vi "Instrument.Lockin.AppLauncher.vi"() -> ()   [LabVIEW 2019, in "Instrument.Lockin.lvlib" / "Instrument.Lockin.lvclass"]
uses:
  Instrument.Lockin.lvclass
  Instrument.Lockin.lvclass/Instrument.Lockin.ctl
  Instrument UI.Lockin/Instrument UI.Lockin.lvclass
  <userlib>/_OpenG.lib/appcontrol/appcontrol.llb/openg_application_control.lvlib
  <userlib>/LevyLab/Instrument Framework/Instrument UI/Instrument UI.lvclass
  <userlib>/LevyLab/Instrument Framework/Instrument/Instrument.lvclass
  <vilib>/numeric/Random Number (Range) U64.vi
  <vilib>/JKI/JKI SMO/SMO/Typedefs/SMOState --Enum.ctl
  <vilib>/JKI/JKI SMO/SMO/SMO.lvclass
  <vilib>/JKI/JKI SMO/SMO.UI/SMO.UI.lvclass
  Lockin.Utilities/Lockin.Utilities.lvlib
panel:
  in  "Examine Configuration.ini":bool
  out "error out":errorcluster
  in  "Splash Status":string="Push Start to Start..." caption="String"
  in  "Debug Mode":bool
  in  "Start Application":bool caption="Play"
  in  "Stop Application":bool caption="Stop"
  out "version":string
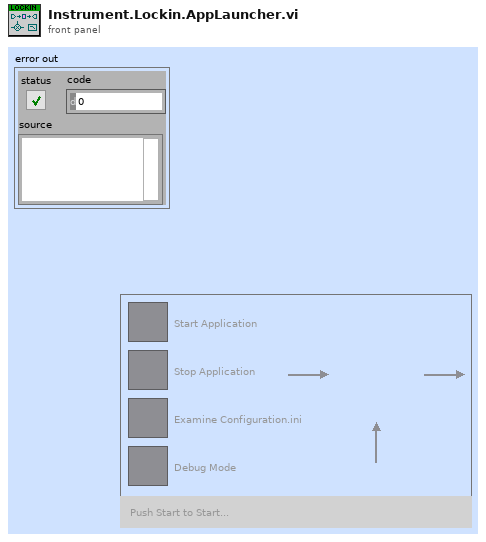
[diagram p1: front panel]
types:
  T1 = typedef "SMO.lvclass/SMOState --Enum.ctl" = enum16{"unknown", "Created", "Started", "Stopped"}
  T2 = enum32{"Invalid", "Standard", "Closed", "Hidden", "Minimized", "Maximized"}
  T3 = enum32{"invalid app kind", "Development System", "Run Time System", "Student Edition", "Embedded LabVIEW", "Evaluation", "Custom"}
  T4 = typedef "SMO.UI.lvclass/SMO.UI State--enum.ctl" = enum16{"unknown", "Opened", "Closed"}
  T5 = cluster{"Core":cluster{"Current VI Reference":refnum<vi>, "Close Panel on Exit?":bool}, "Instrument.Lockin":refnum<class "Instrument.Lockin.lvclass">, "Instrument UI.Lockin":refnum<class "Instrument UI.Lockin.lvclass">}
  T6 = cluster{"Current VI Reference":refnum<vi>, "Close Panel on Exit?":bool}
  T7 = typedef "SMO.lvclass/Public Events.ctl" = cluster{"Error":refnum<user-event>, "State":refnum<user-event>, "Reserve State":refnum<user-event>}
  T8 = typedef "SMO.UI.lvclass/PublicEvents--Cluster.ctl" = cluster{"UI Hidden":refnum<user-event>, "UI State":refnum<user-event>}
  T9 = cluster{"Event Registration Refnum":refnum<event-registration>, "Event Registration Refnum":refnum<event-registration>}
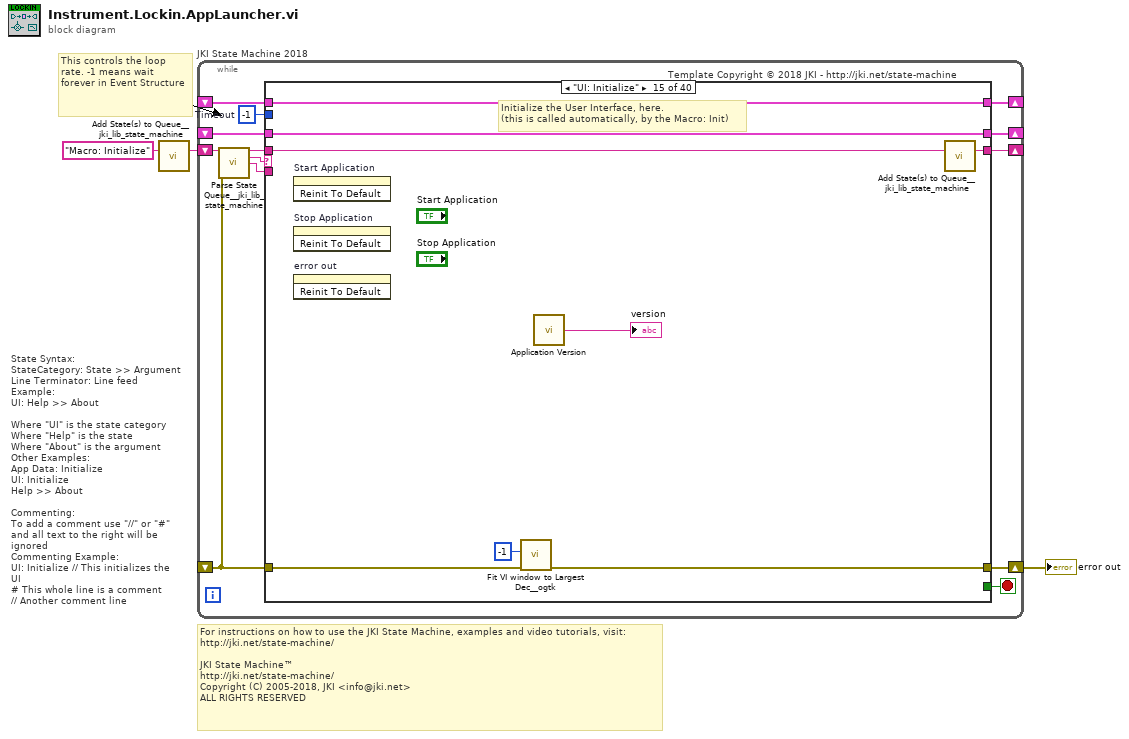
[diagram p0: block diagram]
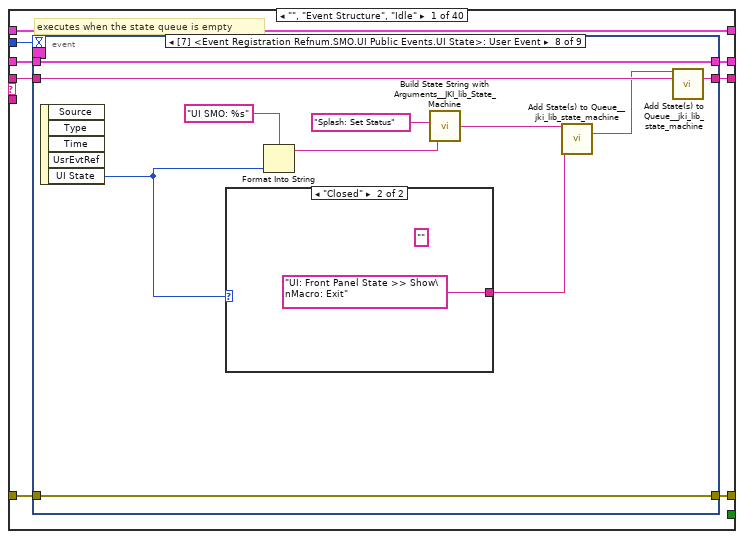
[diagram p2: hidden frame]
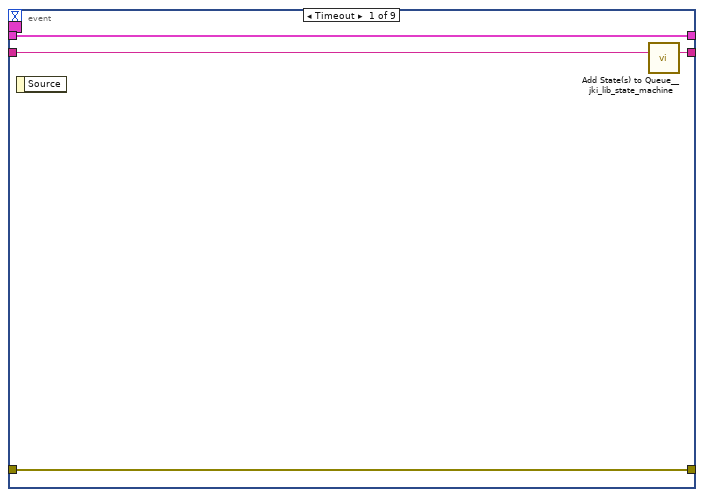
[diagram p3: hidden frame]
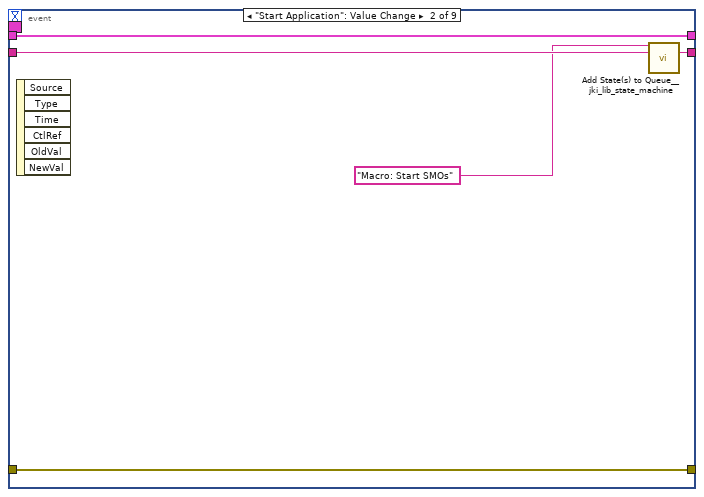
[diagram p4: hidden frame]
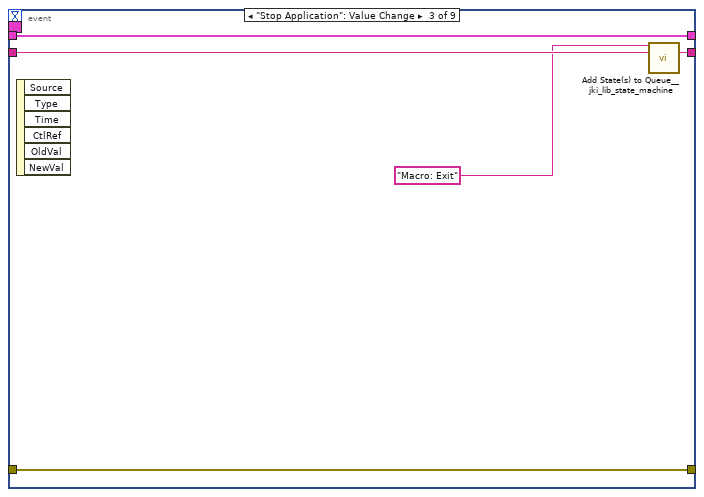
[diagram p5: hidden frame]
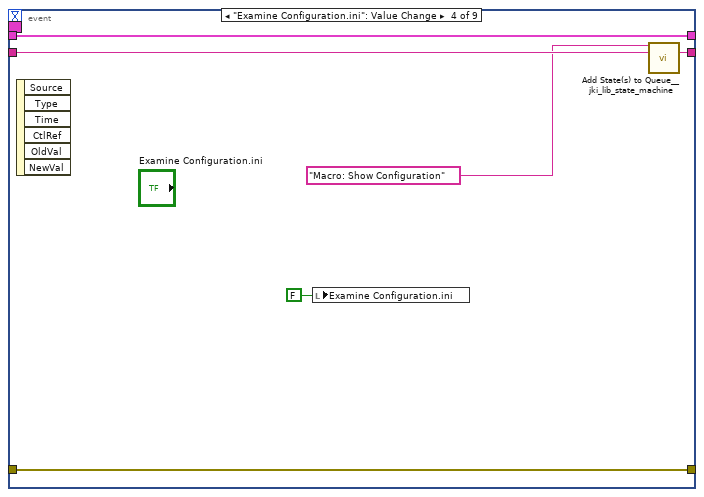
[diagram p6: hidden frame]
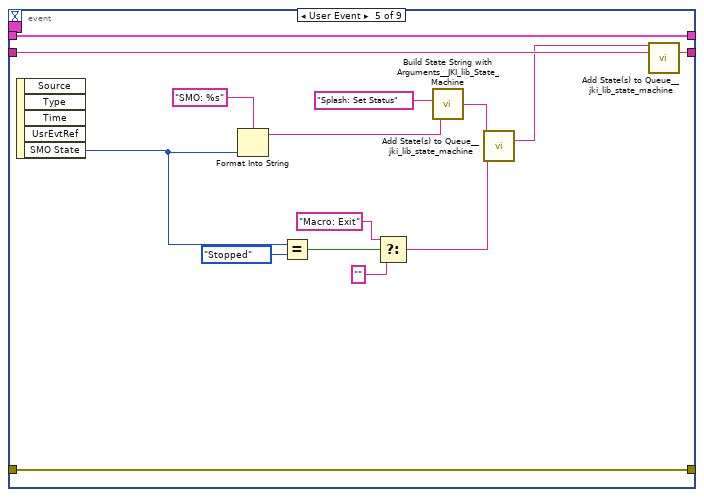
[diagram p7: hidden frame]
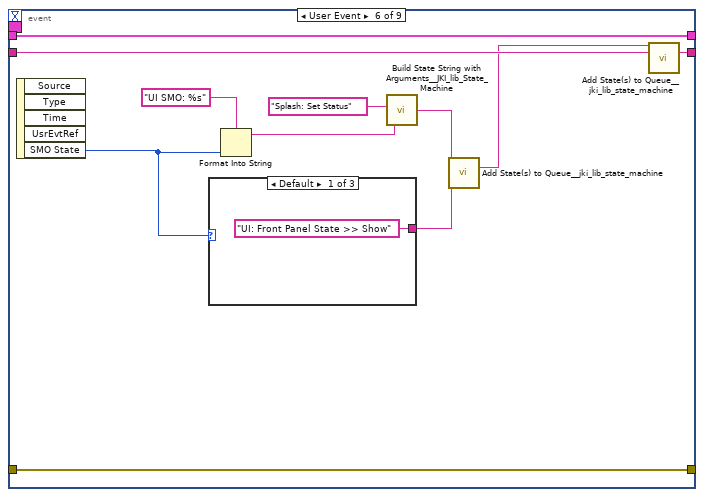
[diagram p8: hidden frame]
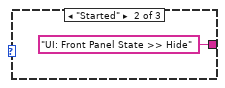
[diagram p9: hidden frame]
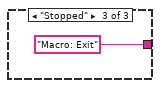
[diagram p10: hidden frame]
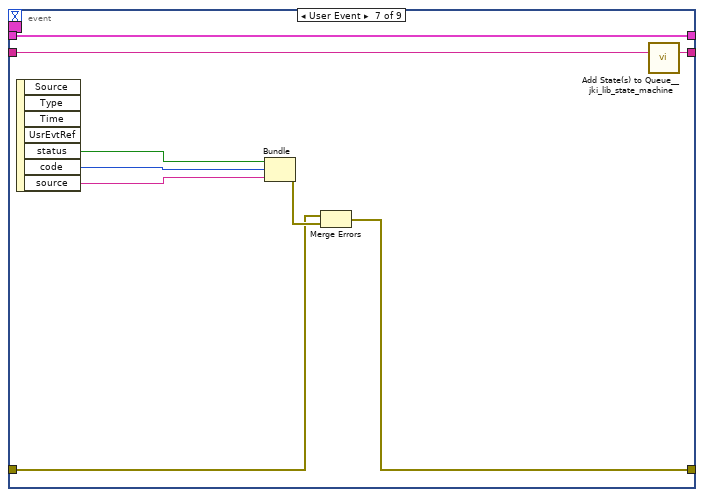
[diagram p11: hidden frame]
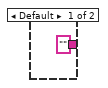
[diagram p12: hidden frame]
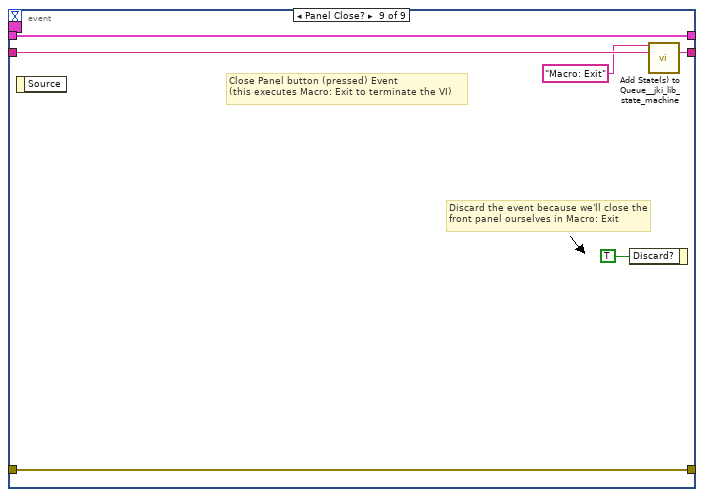
[diagram p13: hidden frame]
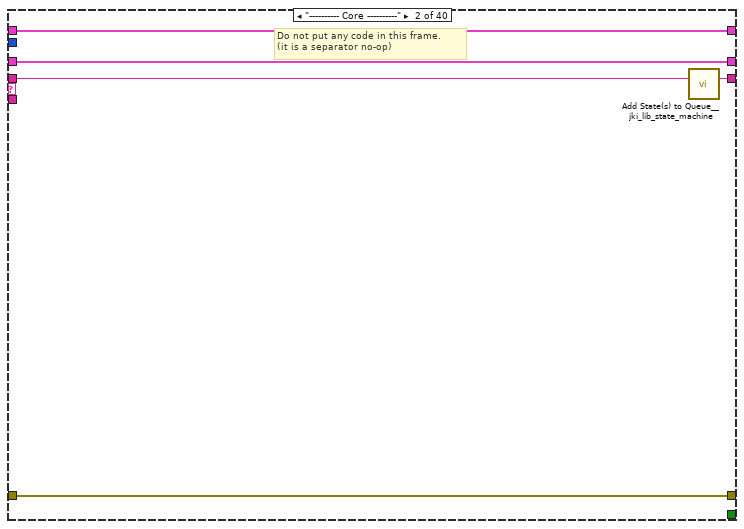
[diagram p14: hidden frame]
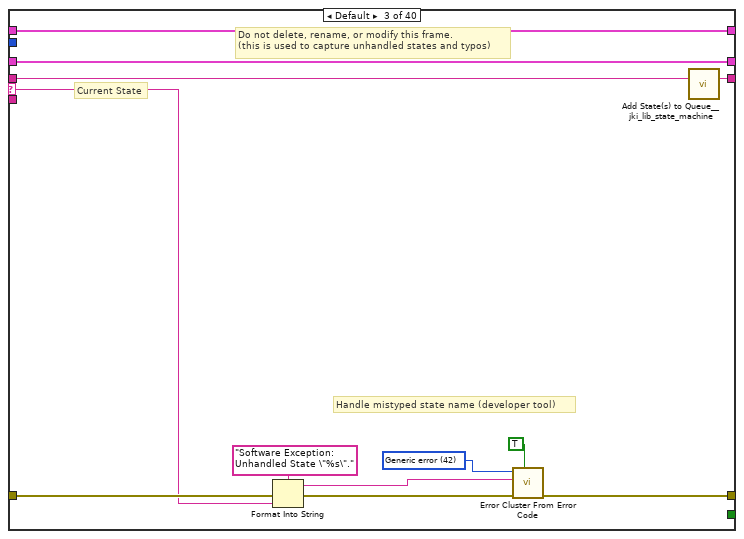
[diagram p15: hidden frame]
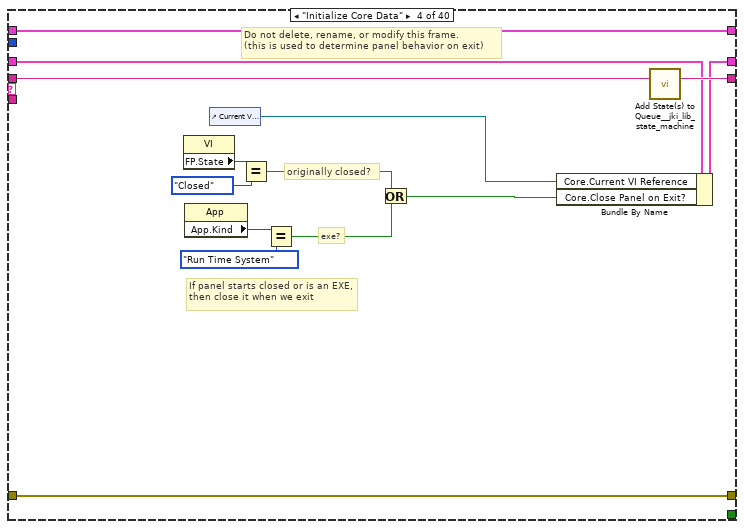
[diagram p16: hidden frame]
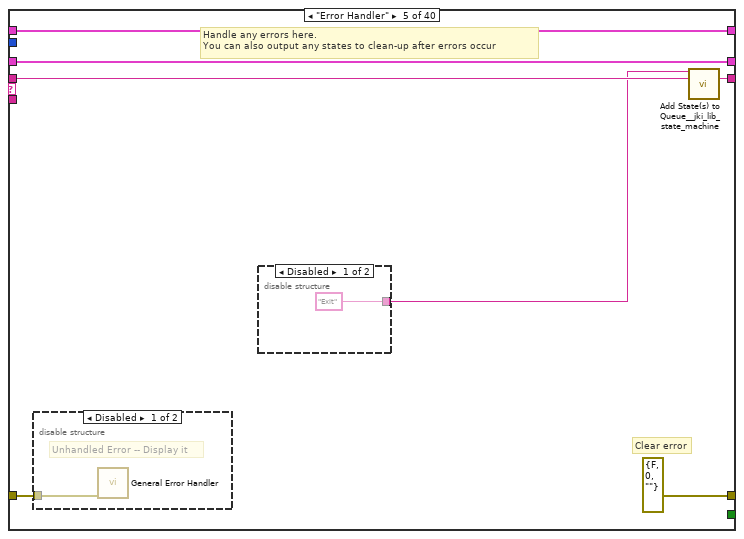
[diagram p17: hidden frame]
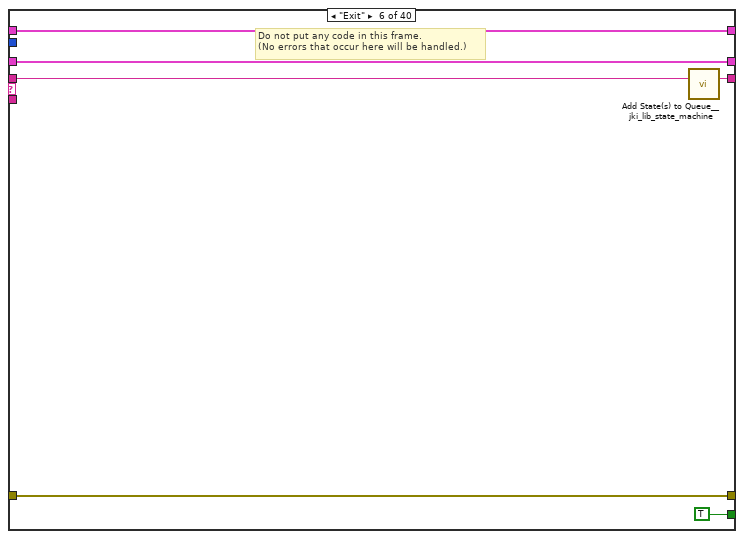
[diagram p20: hidden frame]
diagram:
  # "For instructions on how to use the JKI State Machine, examples and video tutorials, visit:\nhttp://jki.net/state-machine/\n\nJKI State Machine™\nhttp://jki.net/state-machine/\nCopyright (C) 2005-2018, JKI <info@jki.net>\nALL RIGHTS RESERVED"
  # "State Syntax:\nStateCategory: State >> Argument\nLine Terminator: Line feed\nExample:\nUI: Help >> About\n\nWhere \"UI\" is the state category\nWhere \"Help\" is the state\nWhere \"About\" is the argument\nOther Examples:\nApp Data: Initialize\nUI: Initialize\nHelp >> About\n\nCommenting:\nTo add a comment use \"//\" or \"#\" and all text to the right will be ignored\nCommenting Example:\nUI: Initialize // This initializes the UI\n# This whole line is a comment\n// Another comment line"
  # "This controls the loop rate. -1 means wait forever in Event Structure"
  n1 = call <vilib>:"Add State(s) to Queue__jki_lib_state_machine.vi"("State(s) in (\"\")"="Macro: Initialize") -> ("States Out"=w3:string)  [unwired: 14 in]
  n2 = while "JKI State Machine 2018" {
    shift-right: [w9] -> _
    shift-left: _ -> [w4]
    shift-right: [w12] -> w1
    shift-left: _ -> [w7]
    shift-right: [w11] -> _
    shift-left: w3 -> [w13]
    shift-right: [w6] -> _
    shift-left: _ -> [w5]
    stop <- w10 stop-if-true
    w8 = -1  # Timeout
    # "Template Copyright © 2018 JKI - http://jki.net/state-machine"
    n3 = call <vilib>:"Parse State Queue__jki_lib_state_machine.vi"("State Queue"=w13, "Error In (no error)"=w7) -> ("Remaining States"=w15:string, "Current State"=w16:string, "Arguments"=w14:string)  [unwired: 11 in]
    n4 = case shown="\"UI: Initialize\"" w16 {
      selector: w16 -> [_ _ w108 _ _ _ _ _ _ _ _ _ _ _ _ _ _ _ _ _ _ _ _ _ _ _ _ _ _ _ _ _ _ _ _ _ _ _ _ _]
      tunnel: w15 -> [w24 w106 w112 w132 w139 w147 w152 w160 w167 w175 w180 w197 w203 w208 w216 w223 w230 w242 w325 w330 w335 w341 w347 w353 w359 w371 w376 w387 w396 w407 w422 w436 w443 w454 w469 w484 w499 w508 w515 w520]
      tunnel: w14 -> [_ _ _ _ _ _ _ _ _ w168 _ _ _ _ _ _ w225 w236 _ _ _ _ _ _ _ _ _ _ _ _ _ _ _ _ _ _ _ _ w512 _]
      tunnel: [w21 w104 w114 w129 errorcluster {"status"=FALSE, "code"=0, "source"=""} ("error out") w144 w150 w157 w163 w173 w178 w182 w198 w206 w211 w218 w226 w239 w316 w328 w333 w339 w345 w351 w357 w369 w374 w380 w388 w404 w418 w430 w437 w450 w465 w481 w496 w506 w510 w518] -> w12
      tunnel: w7 -> [w20 w104 w113 w129 w135 w144 w150 w157 w164 w173 w178 w181 w199 w206 w213 w217 w227 w240 w317 w328 w333 w339 w345 w351 w357 w369 w374 w377 w389 w402 w414 w429 w438 w447 w462 w479 w492 w506 w511 w518]
      tunnel: [w23 w105 w111 w131 w138 w146 w151 w159 w166 w174 w179 w196 w202 w207 w215 w222 w229 w241 w324 w329 w334 w340 w346 w352 w358 w370 w375 w386 w395 w406 w421 w435 w442 w453 w468 w483 w498 w507 w514 w519] -> w11
      tunnel: [_ _ _ _ _ TRUE _ _ _ _ _ _ _ _ _ _ _ _ _ _ _ _ _ _ _ _ _ _ _ _ _ _ _ _ _ _ _ _ _ _] -> w10
      tunnel: [w19 w103 w110 w130 w136 w145 w149 w158 w161 w172 w177 w191 w201 w205 w214 w219 w228 w238 w314 w327 w332 w338 w344 w350 w356 w368 w373 w384 w391 w403 w419 w432 w440 w451 w466 w480 w495 w505 w513 w517] -> w9
      tunnel: w8 -> [w18 _ _ _ _ _ _ _ _ _ _ _ _ _ _ _ _ _ _ _ _ _ _ _ _ _ _ _ _ _ _ _ _ _ _ _ _ _ _ _]
      tunnel: [w17 w102 w107 w119 w133 w142 w148 w155 w162 w171 w176 w194 w200 w204 w212 w221 w224 w235 w315 w326 w331 w336 w342 w349 w355 w362 w372 w385 w394 w405 w420 w434 w441 w452 w467 w482 w497 w504 w509 w516] -> w6
      tunnel: w5 -> [w17 w102 w107 w119 w133 w142 w148 w155 w162 w171 w176 _ w200 w204 w212 w221 w224 w235 w315 w326 w331 w336 w342 w349 w355 w362 w372 w385 w394 w405 w420 w434 w441 w452 w467 w482 w497 w504 w509 w516]
      tunnel: w4 -> [w22 w103 w110 w125 w136 w145 w149 _ w161 w172 w177 w191 w201 w205 w214 w219 w228 w238 w314 w327 w332 w338 w344 w350 w356 w368 w373 w379 w392 w403 w419 w433 w440 w451 w466 w480 w495 w505 w513 w517]
      frame "", "Event Structure", "Idle" {
        # "executes when the state queue is empty"
        n5 = event shown="[7] <Event Registration Refnum.SMO.UI Public Events.UI State>: User Event" {
          selector: w17 -> [_ _ _ _ _ _ _ _ _]
          dyn-events: _ -> [_ _ _ _ _ _ _ _ _]
          timeout: w18 -> [_ _ _ _ _ _ _ _ _]
          tunnel: w24 -> [w28 w33 w38 w44 w59 w70 w82 w93 w101]
          tunnel: [w27 w32 w37 w43 w58 w69 w81 w92 w100] -> w23
          tunnel: w22 -> [w25 w30 w35 w41 w56 w67 w80 w91 w98]
          tunnel: [w26 w31 w36 w42 w57 w68 w77 w90 w99] -> w21
          tunnel: w20 -> [w26 w31 w36 w42 w57 w68 w78 w90 w99]
          tunnel: [w25 w30 w35 w41 w56 w67 w80 w91 w98] -> w19
          event Timeout {
            n6 = event-data() -> ()  [unwired: 1 in, 1 out]
            n7 = call <vilib>:"Add State(s) to Queue__jki_lib_state_machine.vi"("State(s) in (\"\")"=w28) -> ("States Out"=w27:string)  [unwired: 14 in]
          }
          event "Start Application": Value Change {
            n8 = event-data() -> ()  [unwired: 1 in, 6 out]
            n9 = call <vilib>:"Add State(s) to Queue__jki_lib_state_machine.vi"("State(s) in Front (\"\")"="Macro: Start SMOs" ("State(s) in Front (\"\")"), "State(s) in (\"\")"=w33) -> ("States Out"=w32:string)  [unwired: 13 in]
          }
          event "Stop Application": Value Change {
            n10 = event-data() -> ()  [unwired: 1 in, 6 out]
            n11 = call <vilib>:"Add State(s) to Queue__jki_lib_state_machine.vi"("State(s) in Front (\"\")"="Macro: Exit" ("State(s) in Front (\"\")"), "State(s) in (\"\")"=w38) -> ("States Out"=w37:string)  [unwired: 13 in]
          }
          event "Examine Configuration.ini": Value Change {
            n12 = event-data() -> ()  [unwired: 1 in, 6 out]
            n13 = local write "Examine Configuration.ini"(FALSE ("Examine Configuration.ini")) -> ()
            n14 = call <vilib>:"Add State(s) to Queue__jki_lib_state_machine.vi"("State(s) in Front (\"\")"="Macro: Show Configuration" ("State(s) in Front (\"\")"), "State(s) in (\"\")"=w44) -> ("States Out"=w43:string)  [unwired: 13 in]
          }
          event User Event {
            n15 = event-data() -> ("SMO State"=w51:T1)  [unwired: 1 in, 4 out]
            n16 = Format Into String(format string="SMO: %s", w51) -> (resulting string=w48:string)  [unwired: 2 in, 1 out]
            n17 = Equal?(x=w51, y=SMOState_--Enum."Stopped") -> (x = y?=w54:bool)
            n18 = Select(t="Macro: Exit", s=w54, f="" ("State(s) in Front (\"\")")) -> (s? t:f=w46:string)
            n19 = call <vilib>:"Build State String with Arguments__JKI_lib_State_Machine.vi"("Arguments (\"\")"=w48, "State"="Splash: Set Status" ("t")) -> ("State with Arguments"=w47:string)  [unwired: 4 in]
            n20 = call <vilib>:"Add State(s) to Queue__jki_lib_state_machine.vi"("State(s) in Front (\"\")"=w47, "State(s) at Back (\"\")"=w46) -> ("States Out"=w45:string)  [unwired: 13 in]
            n21 = call <vilib>:"Add State(s) to Queue__jki_lib_state_machine.vi"("State(s) in Front (\"\")"=w45, "State(s) in (\"\")"=w59) -> ("States Out"=w58:string)  [unwired: 13 in]
          }
          event User Event {
            n22 = event-data() -> ("SMO State"=w60:T1)  [unwired: 1 in, 4 out]
            n23 = case shown="Default" w60 {
              tunnel: ["UI: Front Panel State >> Show" ("t") "UI: Front Panel State >> Hide" ("t") "Macro: Exit" ("t")] -> w61
              frame Default {
              }
              frame "Started" {
              }
              frame "Stopped" {
              }
            }
            n24 = Format Into String(format string="UI SMO: %s", w60) -> (resulting string=w64:string)  [unwired: 2 in, 1 out]
            n25 = call <vilib>:"Build State String with Arguments__JKI_lib_State_Machine.vi"("Arguments (\"\")"=w64, "State"="Splash: Set Status" ("t")) -> ("State with Arguments"=w62:string)  [unwired: 4 in]
            n26 = call <vilib>:"Add State(s) to Queue__jki_lib_state_machine.vi"("State(s) in Front (\"\")"=w62, "State(s) at Back (\"\")"=w61) -> ("States Out"=w63:string)  [unwired: 13 in]
            n27 = call <vilib>:"Add State(s) to Queue__jki_lib_state_machine.vi"("State(s) in Front (\"\")"=w63, "State(s) in (\"\")"=w70) -> ("States Out"=w69:string)  [unwired: 13 in]
          }
          event User Event {
            n28 = event-data() -> ("status"=w74:bool, "code"=w76:i32, "source"=w75:string)  [unwired: 1 in, 4 out]
            n29 = Bundle("status"=w74, "code"=w76, "source"=w75) -> (w79:errorcluster)  [unwired: 1 in]
            n30 = Merge Errors(w78, w79) -> (w77:errorcluster)
            n31 = call <vilib>:"Add State(s) to Queue__jki_lib_state_machine.vi"("State(s) in (\"\")"=w82) -> ("States Out"=w81:string)  [unwired: 14 in]
          }
          event User Event {
            n32 = event-data() -> ("UI State"=w86:T4)  [unwired: 1 in, 4 out]
            n33 = case shown="\"Closed\"" w86 {
              tunnel: ["" "UI: Front Panel State >> Show\nMacro: Exit"] -> w84
              frame Default {
              }
              frame "Closed" {
                (unwired) "" ("t")
              }
            }
            n34 = Format Into String(format string="UI SMO: %s", w86) -> (resulting string=w87:string)  [unwired: 2 in, 1 out]
            n35 = call <vilib>:"Build State String with Arguments__JKI_lib_State_Machine.vi"("Arguments (\"\")"=w87, "State"="Splash: Set Status" ("t")) -> ("State with Arguments"=w85:string)  [unwired: 4 in]
            n36 = call <vilib>:"Add State(s) to Queue__jki_lib_state_machine.vi"("State(s) in Front (\"\")"=w85, "State(s) at Back (\"\")"=w84) -> ("States Out"=w83:string)  [unwired: 13 in]
            n37 = call <vilib>:"Add State(s) to Queue__jki_lib_state_machine.vi"("State(s) in Front (\"\")"=w83, "State(s) in (\"\")"=w93) -> ("States Out"=w92:string)  [unwired: 13 in]
          }
          event Panel Close? {
            # "Discard the event because we'll close the front panel ourselves in Macro: Exit"
            # "Close Panel button (pressed) Event\n(this executes Macro: Exit to terminate the VI)"
            n38 = event-data() -> ()  [unwired: 1 in, 1 out]
            n39 = event-data("Discard?"=TRUE) -> ()  [unwired: 1 in, 1 out]
            n40 = call <vilib>:"Add State(s) to Queue__jki_lib_state_machine.vi"("State(s) in Front (\"\")"="Macro: Exit", "State(s) in (\"\")"=w101) -> ("States Out"=w100:string)  [unwired: 13 in]
          }
        }
      }
      frame "---------- Core ----------" {
        # "Do not put any code in this frame.\n(it is a separator no-op)"
        n41 = call <vilib>:"Add State(s) to Queue__jki_lib_state_machine.vi"("State(s) in (\"\")"=w106) -> ("States Out"=w105:string)  [unwired: 14 in]
      }
      frame Default {
        w117 = 42 items=["No error", "Argument error", "Memory is full", "Out of zone", "End of file", "File already open", "Generic file I/O error", "File not found", "File permission error", "Disk is full", "Duplicate path", "Too many files open", "System feature not enabled", "Resource file not found", "Cannot add resource", "Resource not found", "Image not found", "Image memory error", "Pen does not exist", "Config type invalid", "Config token not found", "Config parse error", "Config memory error", "Bad external code format", "Bad external code offset", "External code not present", "Null window", "Destroy window error", "Null menu", "Print aborted", "Bad print record", "Print driver error", "Windows error during printing", "Memory error during printing", "Print dialog error", "Generic print error", "Invalid device refnum", "Device not found", "Device parameter error", "Device unit error", "Cannot open device", "Device call aborted", "Generic error", "Cancelled by user", "Object ID too low", "Object ID too high", "Object not in heap", "Unknown heap", "Unknown object (invalid DefProc)", "Unknown object (DefProc not in table)", "Message out of range", "Invalid (null) method", "Unknown message", "Manager call not supported", "Bad address", "Network operation in progress", "Network operation timed out", "Connection is busy", "Network attribute not supported", "Network error", "Address in use", "System out of memory", "Connection aborted", "Connection refused", "Not connected", "Already connected", "Connection closed", "Initialization error (interapplication manager)", "Bad occurrence", "Wait on unbound occurrence handler", "Occurrence queue overflow", "Datalog type conflict", "Unused", "Unrecognized type (interapplication manager)", "Memory corrupt", "Failed to make temporary DLL", "Old CIN version", "Drag socket not found", "Failed to load drop-object", "Failed to register OLE object", "Failed to release OLE object", "Format specifier type mismatch", "Unknown format specifier", "Too few format specifiers", "Too many format specifiers", "Scan failed", "Newer CIN version", "Error converting to variant", "Runtime menu error", "Password tampered", "Variant attribute not found", "Incompatible variant data type", "Event data is not available", "Event Store is not present", "Occurrence is not found", "Event Queue is not created", "Event info is not available", "Refnum passed is NULL", "Error retrieving Class GUID", "Error retrieving CoClass GUID", "Error retrieving TypeLib GUID.", "Bad built application magic bytes.", "Specific driver is different from the specific driver associated with the Logical Name.", "There is no session opened to the class driver.", "Max Error", "MAX - Error with config objects", "MAX - Error loading configuration", "MAX - Group not supported"]
        # "Current State"
        # "Do not delete, rename, or modify this frame.\n(this is used to capture unhandled states and typos)"
        # "Handle mistyped state name (developer tool)"
        n42 = Format Into String(format string="Software Exception: Unhandled State \"%s\"." ("message"), error in=w113, w108) -> (resulting string=w116:string, error out=w115:errorcluster)  [unwired: 1 in]
        n43 = call <vilib>:"Error Cluster From Error Code.vi"("show call chain? (False)"=TRUE, "error in (no error)"=w115, "error message (\"\")"=w116, "error code (0)"=w117) -> ("error out"=w114:errorcluster)  [unwired: 5 in]
        n44 = call <vilib>:"Add State(s) to Queue__jki_lib_state_machine.vi"("State(s) in (\"\")"=w112) -> ("States Out"=w111:string)  [unwired: 14 in]
      }
      frame "Initialize Core Data" {
        # "Do not delete, rename, or modify this frame.\n(this is used to determine panel behavior on exit)"
        # "originally closed?"
        # "exe?"
        # "If panel starts closed or is an EXE, then close it when we exit"
        n45 = property class="VI"() -> ("FP.State"=w122:T2)  [unwired: 2 in, 2 out]
        n46 = property class="App"() -> ("App.Kind"=w128:T3)  [unwired: 2 in, 2 out]
        n47 = control-ref of="Current VI Reference"() -> (w123:refnum<vi>)
        n48 = Equal?(x=w122, y=T2."Closed" ("Front Panel Window:State")) -> (x = y?=w120:bool)
        n49 = Equal?(x=w128, y=T3."Run Time System" ("Application:Kind")) -> (x = y?=w126:bool)
        n50 = Or(x=w120, y=w126) -> (x .or. y?=w124:bool)
        n51 = Bundle By Name(cluster=w125, "Core.Current VI Reference"=w123, "Core.Close Panel on Exit?"=w124) -> (w130:T5)
        n52 = call <vilib>:"Add State(s) to Queue__jki_lib_state_machine.vi"("State(s) in (\"\")"=w132) -> ("States Out"=w131:string)  [unwired: 14 in]
      }
      frame "Error Handler" {
        # "Handle any errors here.\nYou can also output any states to clean-up after errors occur"
        # "Clear error"
        n53 = disable-structure shown="Disabled" {
          disable-tunnel: w135 -> [w141 _]
          frame Disabled {
            # "Unhandled Error -- Display it"
            n54 = call <vilib>:"General Error Handler.vi"("error in (no error)"=w141) -> ()  [unwired: 10 in, 5 out]
          }
          frame Enabled {
          }
        }
        n55 = disable-structure shown="Disabled" {
          disable-tunnel: ["Exit" _] -> w134
          frame Disabled {
          }
          frame Enabled {
          }
        }
        n56 = call <vilib>:"Add State(s) to Queue__jki_lib_state_machine.vi"("State(s) in Front (\"\")"=w134, "State(s) in (\"\")"=w139) -> ("States Out"=w138:string)  [unwired: 13 in]
      }
      frame "Exit" {
        # "Do not put any code in this frame.\n(No errors that occur here will be handled.)"
        n57 = call <vilib>:"Add State(s) to Queue__jki_lib_state_machine.vi"("State(s) in (\"\")"=w147) -> ("States Out"=w146:string)  [unwired: 14 in]
      }
      frame "---------- Data ----------" {
        # "Do not put any code in this frame.\n(It is a separator no-op. You can make a copy of this frame to create a new Data frame)"
        n58 = call <vilib>:"Add State(s) to Queue__jki_lib_state_machine.vi"("State(s) in (\"\")"=w152) -> ("States Out"=w151:string)  [unwired: 14 in]
      }
      frame "Data: Initialize" {
        w154 = refnum<class "Instrument UI.Lockin.lvclass"> refnum  # Instrument UI.Lockin
        w153 = refnum<class "Instrument.Lockin.lvclass"> refnum  # Instrument.Lockin
        w156 = T6 {"Current VI Reference"=refnum, "Close Panel on Exit?"=FALSE}  # Core
        # "Initialize the shift-register data, here.\n(data names are defined by what you wire into the bundle function)"
        n59 = Bundle("Core"=w156, "Instrument.Lockin"=w153, "Instrument UI.Lockin"=w154) -> (w158:T5)  [unwired: 1 in]
        n60 = call <vilib>:"Add State(s) to Queue__jki_lib_state_machine.vi"("State(s) in (\"\")"=w160) -> ("States Out"=w159:string)  [unwired: 14 in]
      }
      frame "Data: Cleanup" {
        # "Cleanup any data and references, here.\n(this is called automatically, by the Macro: Exit)"
        n61 = Unbundle By Name(w161) -> ("Core.Current VI Reference"=w165:refnum<vi>)
        n62 = Close Reference(reference=w165, error in (no error)=w164) -> (error out=w163:errorcluster)
        n63 = call <vilib>:"Add State(s) to Queue__jki_lib_state_machine.vi"("State(s) in (\"\")"=w167) -> ("States Out"=w166:string)  [unwired: 14 in]
      }
      frame "Data: Wait" {
        # "Do not put any code in this frame.\n(It is a separator no-op. You can make a copy of this frame to create a new Data frame)"
        n64 = Scan From String(input string=w168, default 1=u32 0) -> (output 1=w169:u32)  [unwired: 3 in, 3 out]
        n65 = Wait (ms)(milliseconds to wait=w169) -> ()  [unwired: 1 out]
        n66 = call <vilib>:"Add State(s) to Queue__jki_lib_state_machine.vi"("State(s) in (\"\")"=w175) -> ("States Out"=w174:string)  [unwired: 14 in]
      }
      frame "---------- Events ----------" {
        # "Do not put any code in this frame.\n(It is a separator no-op. You can make a copy of this frame to create a new UI frame)"
        n67 = call <vilib>:"Add State(s) to Queue__jki_lib_state_machine.vi"("State(s) in (\"\")"=w180) -> ("States Out"=w179:string)  [unwired: 14 in]
      }
      frame "Events: Register" {
        # "Do not put any code in this frame.\n(It is a separator no-op. You can make a copy of this frame to create a new UI frame)"
        n68 = Unbundle By Name(w191) -> ("Instrument.Lockin"=w190:refnum<class "Instrument.Lockin.lvclass">, "Instrument UI.Lockin"=w189:refnum<class "Instrument UI.Lockin.lvclass">)
        n69 = call <vilib>:"GetPublicEvents.vi"("SMO"=w190) -> ("error out"=w184:errorcluster, "Public Events"=w192:T7)  [unwired: 8 in, 1 out]
        n70 = call <vilib>:"GetPublicEvents.vi"("SMO"=w189) -> ("error out"=w183:errorcluster, "Public Events"=w193:T7, "SMO out"=w187:refnum<class "Instrument UI.Lockin.lvclass">)  [unwired: 8 in]
        n71 = register-events(w192) -> (reference out=w195:refnum<event-registration>)  [unwired: 2 in, 1 out]
        n72 = call <vilib>:"SMO.UI.GetPublicEvents.vi"("SMO.UI"=w187) -> ("error out"=w185:errorcluster, "SMO.UI Public Events"=w186:T8)  [unwired: 8 in, 1 out]
        n73 = register-events(w193, w186) -> (reference out=w188:refnum<event-registration>)  [unwired: 2 in, 1 out]
        n74 = Merge Errors(w185, w183, w184, w181) -> (w182:errorcluster)
        n75 = Bundle("Event Registration Refnum"=w195, "Event Registration Refnum"=w188) -> (w194:T9)  [unwired: 1 in]
        n76 = call <vilib>:"Add State(s) to Queue__jki_lib_state_machine.vi"("State(s) in (\"\")"=w197) -> ("States Out"=w196:string)  [unwired: 14 in]
      }
      frame "Events: Unregister" {
        # "Do not put any code in this frame.\n(It is a separator no-op. You can make a copy of this frame to create a new UI frame)"
        n77 = Unregister For Events(event registration refnum=w200, error in=w199) -> (error out=w198:errorcluster)
        n78 = call <vilib>:"Add State(s) to Queue__jki_lib_state_machine.vi"("State(s) in (\"\")"=w203) -> ("States Out"=w202:string)  [unwired: 14 in]
      }
      frame "---------- UI ----------" {
        # "Do not put any code in this frame.\n(It is a separator no-op. You can make a copy of this frame to create a new UI frame)"
        n79 = call <vilib>:"Add State(s) to Queue__jki_lib_state_machine.vi"("State(s) in (\"\")"=w208) -> ("States Out"=w207:string)  [unwired: 14 in]
      }
      frame "UI: Initialize" {
        # "Initialize the User Interface, here.\n(this is called automatically, by the Macro: Init)"
        n80 = invoke on="Start Application" class="Bool" method="Reinit To Default"() -> ()  [unwired: 3 in, 3 out]
        n81 = invoke on="Stop Application" class="Bool" method="Reinit To Default"() -> ()  [unwired: 3 in, 3 out]
        n82 = invoke on="error out" class="Clust (strict)" method="Reinit To Default"() -> ()  [unwired: 3 in, 3 out]
        n83 = call <userlib>:"Fit VI window to Largest Dec__ogtk.vi"("error in (no error)"=w213, "border spacing (2 px)"=-1) -> ("error out"=w211:errorcluster)  [unwired: 4 in, 1 out]
        n84 = call "Application Version.vi"() -> ("Version"=→"version":string)
        n85 = call <vilib>:"Add State(s) to Queue__jki_lib_state_machine.vi"("State(s) in (\"\")"=w216) -> ("States Out"=w215:string)  [unwired: 14 in]
      }
      frame "UI: Open Configuration.ini" {
        # "Do not put any code in this frame.\n(It is a separator no-op. You can make a copy of this frame to create a new UI frame)"
        n86 = Unbundle By Name(w219) -> ("Instrument.Lockin"=w220:refnum<class "Instrument.Lockin.lvclass">)
        n87 = call <userlib>:"Examine Configuration.vi"("error in (no error)"=w217, "Instrument in"=w220) -> ("error out"=w218:errorcluster)  [unwired: 8 in, 1 out]
        n88 = call <vilib>:"Add State(s) to Queue__jki_lib_state_machine.vi"("State(s) in (\"\")"=w223) -> ("States Out"=w222:string)  [unwired: 14 in]
      }
      frame "UI: Cursor Set" {
        # "Argument"
        # "Set and Unset Cursor Busy.\n(Usage: \"UI: Cursor Set >> Busy|Idle\")"
        n89 = case shown="\"Busy\"" w225 {
          tunnel: w227 -> [w232 w234]
          tunnel: [w231 w233] -> w226
          frame "Idle", Default {
            n90 = call <vilib>:"Unset Busy.vi"("error in (no error)"=w232) -> ("error out"=w231:errorcluster)  [unwired: 10 in]
          }
          frame "Busy" {
            n91 = call <vilib>:"Set Busy.vi"("error in (no error)"=w234) -> ("error out"=w233:errorcluster)  [unwired: 9 in, 1 out]
          }
        }
        n92 = call <vilib>:"Add State(s) to Queue__jki_lib_state_machine.vi"("State(s) in (\"\")"=w230) -> ("States Out"=w229:string)  [unwired: 14 in]
      }
      frame "UI: Front Panel State" {
        # "Argument"
        # "Set Front Panel Open or Closed\n(Usage: \"UI: Front Panel State >> Open|Close\")"
        n93 = Unbundle By Name(w238) -> ("Core.Current VI Reference"=w237:refnum<vi>)
        n94 = case shown="\"Open\", \"Standard\", Default" w236 {
          tunnel: w240 -> [w248 w263 w274 w287 w300]
          tunnel: [w250 w264 w276 w289 w302] -> w239
          tunnel: w237 -> [w249 w261 w275 w288 w301]
          frame "Open", "Standard", Default {
            w243 = T2."Standard" ("State")
            n95 = property class="VI"(reference=w249, error in=w248) -> (reference out=w246:refnum<vi>, error out=w247:errorcluster, "FP.State"=w245:T2)
            n96 = Not Equal?(x=w245, y=w243) -> (x != y?=w244:bool)
            n97 = case shown="False" w244 {
              tunnel: [w254 w256] -> w250
              tunnel: w247 -> [w253 w256]
              tunnel: w246 -> [w252 _]
              tunnel: w243 -> [w251 _]
              frame True {
                n98 = invoke class="VI" method="FP.Open"(reference=w252, error in=w253, "Activate"=TRUE, "State"=w251) -> (error out=w254:errorcluster)  [unwired: 1 in, 4 out]
              }
              frame False {
              }
            }
          }
          frame "Close", "Closed" {
            n99 = property class="VI"(reference=w261, error in=w263) -> (reference out=w260:refnum<vi>, error out=w262:errorcluster, "FP.State"=w258:T2)
            n100 = Not Equal?(x=w258, y=T2."Closed" ("Front Panel Window:State")) -> (x != y?=w257:bool)
            n101 = case shown="True" w257 {
              tunnel: [w265 w268] -> w264
              tunnel: w262 -> [w265 w267]
              tunnel: w260 -> [_ w266]
              frame False {
              }
              frame True {
                n102 = invoke class="VI" method="FP.Close"(reference=w266, error in=w267) -> (error out=w268:errorcluster)  [unwired: 1 in, 2 out]
              }
            }
          }
          frame "Hidden", "Hide" {
            w269 = T2."Hidden" ("State")
            n103 = property class="VI"(reference=w275, error in=w274) -> (reference out=w272:refnum<vi>, error out=w273:errorcluster, "FP.State"=w271:T2)
            n104 = Not Equal?(x=w271, y=w269) -> (x != y?=w270:bool)
            n105 = case shown="True" w270 {
              tunnel: [w280 w281] -> w276
              tunnel: w273 -> [w279 w281]
              tunnel: w272 -> [w278 _]
              tunnel: w269 -> [w277 _]
              frame True {
                n106 = invoke class="VI" method="FP.Open"(reference=w278, error in=w279, "State"=w277) -> (error out=w280:errorcluster)  [unwired: 2 in, 4 out]
              }
              frame False {
              }
            }
          }
          frame "Minimize", "Minimized" {
            w282 = T2."Minimized" ("State")
            n107 = property class="VI"(reference=w288, error in=w287) -> (reference out=w285:refnum<vi>, error out=w286:errorcluster, "FP.State"=w284:T2)
            n108 = Not Equal?(x=w284, y=w282) -> (x != y?=w283:bool)
            n109 = case shown="True" w283 {
              tunnel: [w293 w294] -> w289
              tunnel: w286 -> [w292 w294]
              tunnel: w285 -> [w291 _]
              tunnel: w282 -> [w290 _]
              frame True {
                n110 = invoke class="VI" method="FP.Open"(reference=w291, error in=w292, "State"=w290) -> (error out=w293:errorcluster)  [unwired: 2 in, 4 out]
              }
              frame False {
              }
            }
          }
          frame "Maximize", "Maximized" {
            w295 = T2."Maximized" ("State")
            n111 = property class="VI"(reference=w301, error in=w300) -> (reference out=w298:refnum<vi>, error out=w299:errorcluster, "FP.State"=w297:T2)
            n112 = Not Equal?(x=w297, y=w295) -> (x != y?=w296:bool)
            n113 = case shown="True" w296 {
              tunnel: [w306 w307] -> w302
              tunnel: w299 -> [w305 w307]
              tunnel: w298 -> [w304 _]
              tunnel: w295 -> [w303 _]
              frame True {
                n114 = invoke class="VI" method="FP.Open"(reference=w304, error in=w305, "State"=w303) -> (error out=w306:errorcluster)  [unwired: 2 in, 4 out]
              }
              frame False {
              }
            }
          }
        }
        n115 = call <vilib>:"Add State(s) to Queue__jki_lib_state_machine.vi"("State(s) in (\"\")"=w242) -> ("States Out"=w241:string)  [unwired: 14 in]
      }
      frame "UI: Set Background Color" {
        # "Do not put any code in this frame.\n(It is a separator no-op. You can make a copy of this frame to create a new UI frame)"
        n116 = property class="VI"(error in=w317) -> (error out=w319:errorcluster, "Panel"=w320:refnum<vi>)  [unwired: 1 in, 1 out]
        n117 = property class="Pnl"(reference=w320, error in=w319) -> (error out=w318:errorcluster, "Panes[]"=w321:refnum<vi>[])  [unwired: 1 out]
        n118 = call-poly <vilib>:"Random Number (Range).vi"("lower bound (0)"=u64 0, "upper bound (100)"=u64 3) -> ("number"=w308:u64)  [unwired: 9 in]
        n119 = To Long Integer(number=w308) -> (32bit integer=w309:i32)
        n120 = Index Array(array=w321, index=0) -> (element=w323:refnum<vi>)
        n121 = Index Array(array=u32[] [16759480, 13624063, 13631444, 16646072] ("Color Box"), index=w309) -> (element=w310:u32)
        n122 = property class="Pane"(reference=w323, error in=w318, "PaneColor"=w310) -> (error out=w316:errorcluster)  [unwired: 1 out]
        n123 = call <vilib>:"Add State(s) to Queue__jki_lib_state_machine.vi"("State(s) in (\"\")"=w325) -> ("States Out"=w324:string)  [unwired: 14 in]
      }
      frame "UI: Exit" {
        # "Do not put any code in this frame.\n(It is a separator no-op. You can make a copy of this frame to create a new UI frame)"
        n124 = invoke on="Start Application" class="Bool" method="Reinit To Default"() -> ()  [unwired: 3 in, 3 out]
        n125 = invoke on="Stop Application" class="Bool" method="Reinit To Default"() -> ()  [unwired: 3 in, 3 out]
        n126 = call <vilib>:"Add State(s) to Queue__jki_lib_state_machine.vi"("State(s) in (\"\")"=w330) -> ("States Out"=w329:string)  [unwired: 14 in]
      }
      frame "---------- Macro ----------" {
        # "Do not put any code in this frame.\n(It is a separator no-op. You can make a copy of this frame to create a new Macro frame)"
        n127 = call <vilib>:"Add State(s) to Queue__jki_lib_state_machine.vi"("State(s) in (\"\")"=w335) -> ("States Out"=w334:string)  [unwired: 14 in]
      }
      frame "Macro: Initialize" {
        # "Initialization Macro\n(This is called once, when the VI starts)"
        n128 = call <vilib>:"Add State(s) to Queue__jki_lib_state_machine.vi"("State(s) in Front (\"\")"="Data: Initialize\nInitialize Core Data\n//Events: Register\nUI: Initialize\nUI: Front Panel State >> Open\nUI: Set Background Color\nSplash: Set Status >> ...", "State(s) in (\"\")"=w341) -> ("States Out"=w340:string)  [unwired: 13 in]
      }
      frame "Macro: Show Configuration" {
        # "Initialization Macro\n(This is called once, when the VI starts)"
        n129 = call <vilib>:"Add State(s) to Queue__jki_lib_state_machine.vi"("State(s) in Front (\"\")"="Splash: Set Status >> Opening Configuration...\nUI: Open Configuration.ini\nData: Wait >> 1000\nSplash: Set Status >> ...", "State(s) in (\"\")"=w347) -> ("States Out"=w346:string)  [unwired: 13 in]
      }
      frame "Macro: Start SMOs" {
        # "Do not put any code in this frame.\n(It is a separator no-op. You can make a copy of this frame to create a new Macro frame)"
        n130 = call <vilib>:"Add State(s) to Queue__jki_lib_state_machine.vi"("State(s) in Front (\"\")"="Splash: Set Status >> Creating Instrument...\nSMO: Create Instrument\nData: Wait >> 100\nSplash: Set Status >> Creating Instrument UI...\nSMO: Create Instrument UI\nData: Wait >> 100\nSplash: Set Status >> Registering Events...\nEvents: Register\nData: Wait >> 100\nSplash: Set Status >> Starting Instrument...\nSMO: Start Instrument\nData: Wait >> 100\nSplash: Set Status >> Instrument Process Started...\nData: Wait >> 100\nSplash: Set Status >> Starting User Interface...\nSMO: Start Instrument UI\nData: Wait >> 100\nUI: Front Panel State >> Hide\nSMO: Show Instrument UI" ("State(s) in Front (\"\")"), "State(s) in (\"\")"=w353) -> ("States Out"=w352:string)  [unwired: 13 in]
      }
      frame "Macro: Stop SMOs" {
        # "Do not put any code in this frame.\n(It is a separator no-op. You can make a copy of this frame to create a new Macro frame)"
        n131 = call <vilib>:"Add State(s) to Queue__jki_lib_state_machine.vi"("State(s) in Front (\"\")"="UI: Front Panel State >> Show\nSplash: Set Status >> Stopping Instrument...\nSMO: Stop Instrument\nData: Wait >> 100\nSplash: Set Status >> Destroying Instrument...\nSMO: Destroy Instrument\nData: Wait >> 100\nSplash: Set Status >>Hiding UI...\nSMO: Hide Instrument UI\nData: Wait >> 100\nSplash: Set Status >> Stopping UI...\nSMO: Stop Instrument UI\nData: Wait >> 100\nSplash: Set Status >> Destroying UI...\nSMO: Destroy Instrument UI" ("State(s) in Front (\"\")"), "State(s) in (\"\")"=w359) -> ("States Out"=w358:string)  [unwired: 13 in]
      }
      frame "Macro: Exit" {
        # "Exit Macro\n(This is called once, when the VI exits)"
        n132 = Unbundle By Name(w368) -> ("Core.Close Panel on Exit?"=w367:bool)
        n133 = Select(t="UI: Front Panel State >> Close", s=w367, f="") -> (s? t:f=w364:string)
        n134 = call <vilib>:"Add State(s) to Queue__jki_lib_state_machine.vi"("State(s) in Front (\"\")"="UI: Front Panel State >> Open\nMacro: Stop SMOs\nUI: Exit", "State(s) in (\"\")"=w364, "State(s) at Back (\"\")"="Data: Cleanup\nEvents: Unregister\nExit") -> ("States Out"=w363:string)  [unwired: 12 in]
        n135 = call <vilib>:"Add State(s) to Queue__jki_lib_state_machine.vi"("State(s) in Front (\"\")"=w363, "State(s) in (\"\")"=w371) -> ("States Out"=w370:string)  [unwired: 13 in]
      }
      frame "---------- SMO ----------" {
        # "Do not put any code in this frame.\n(It is a separator no-op. You can make a copy of this frame to create a new Macro frame)"
        n136 = call <vilib>:"Add State(s) to Queue__jki_lib_state_machine.vi"("State(s) in (\"\")"=w376) -> ("States Out"=w375:string)  [unwired: 14 in]
      }
      frame "SMO: Create Instrument" {
        # "Do not put any code in this frame.\n(It is a separator no-op. You can make a copy of this frame to create a new Macro frame)"
        n137 = Unbundle By Name(w379) -> ("Instrument.Lockin"=w378:refnum<class "Instrument.Lockin.lvclass">)
        n138 = call <userlib>:"Create Instrument SMO.vi"("error in (no error)"=w377, "Debug Mode? [F]"="Debug Mode", "Configuration Window? [T]"=FALSE, "Instrument in"=w378) -> ("error out"=w380:errorcluster, "Instrument out"=w381:refnum<class "Instrument.Lockin.lvclass">)  [unwired: 6 in]
        n139 = Bundle By Name(cluster=w379, "Instrument.Lockin"=w381) -> (w384:T5)
        n140 = call <vilib>:"Add State(s) to Queue__jki_lib_state_machine.vi"("State(s) in (\"\")"=w387) -> ("States Out"=w386:string)  [unwired: 14 in]
      }
      frame "SMO: Start Instrument" {
        # "Do not put any code in this frame.\n(It is a separator no-op. You can make a copy of this frame to create a new Macro frame)"
        n141 = Unbundle By Name(w392) -> ("Instrument.Lockin"=w393:refnum<class "Instrument.Lockin.lvclass">)
        n142 = call <vilib>:"Start.vi"("error in (no error)"=w389, "SMO"=w393) -> ("error out"=w388:errorcluster, "SMO out"=w390:refnum<class "Instrument.Lockin.lvclass">)  [unwired: 8 in]
        n143 = Bundle By Name(cluster=w392, "Instrument.Lockin"=w390) -> (w391:T5)
        n144 = call <vilib>:"Add State(s) to Queue__jki_lib_state_machine.vi"("State(s) in (\"\")"=w396) -> ("States Out"=w395:string)  [unwired: 14 in]
      }
      frame "SMO: Stop Instrument" {
        # "Do not put any code in this frame.\n(It is a separator no-op. You can make a copy of this frame to create a new Macro frame)"
        n145 = Unbundle By Name(w403) -> ("Instrument.Lockin"=w398:refnum<class "Instrument.Lockin.lvclass">)
        n146 = call <vilib>:"GetState.vi"("error in (no error)"=w402, "SMO"=w398) -> ("error out"=w401:errorcluster, "SMO State"=w399:T1, "SMO out"=w397:refnum<class "Instrument.Lockin.lvclass">)  [unwired: 7 in]
        n147 = call <vilib>:"Clear Errors.vi"("error in (no error)"=w401) -> ("error out"=w400:errorcluster)  [unwired: 5 in, 1 out]
        n148 = case shown="\"Created\", \"Started\"" w399 {
          tunnel: [w408 w411] -> w404
          tunnel: w397 -> [_ w410]
          tunnel: w400 -> [w408 w409]
          frame Default {
          }
          frame "Created", "Started" {
            n149 = call <vilib>:"Stop.vi"("error in (no error)"=w409, "SMO"=w410) -> ("error out"=w411:errorcluster)  [unwired: 8 in, 1 out]
          }
        }
        n150 = call <vilib>:"Add State(s) to Queue__jki_lib_state_machine.vi"("State(s) in (\"\")"=w407) -> ("States Out"=w406:string)  [unwired: 14 in]
      }
      frame "SMO: Destroy Instrument" {
        # "Do not put any code in this frame.\n(It is a separator no-op. You can make a copy of this frame to create a new Macro frame)"
        n151 = Unbundle By Name(w419) -> ("Instrument.Lockin"=w417:refnum<class "Instrument.Lockin.lvclass">)
        n152 = call <vilib>:"GetState.vi"("error in (no error)"=w414, "SMO"=w417) -> ("error out"=w413:errorcluster, "SMO State"=w416:T1, "SMO out"=w412:refnum<class "Instrument.Lockin.lvclass">)  [unwired: 7 in]
        n153 = call <vilib>:"Clear Errors.vi"("error in (no error)"=w413) -> ("error out"=w415:errorcluster)  [unwired: 5 in, 1 out]
        n154 = case shown="\"Stopped\"" w416 {
          tunnel: [w423 w426] -> w418
          tunnel: w415 -> [w423 w425]
          tunnel: w412 -> [_ w424]
          frame Default {
          }
          frame "Stopped" {
            n155 = call <vilib>:"Destroy.vi"("error in (no error)"=w425, "SMO"=w424) -> ("error out"=w426:errorcluster)  [unwired: 9 in]
          }
        }
        n156 = call <vilib>:"Add State(s) to Queue__jki_lib_state_machine.vi"("State(s) in (\"\")"=w422) -> ("States Out"=w421:string)  [unwired: 14 in]
      }
      frame "SMO: Create Instrument UI" {
        # "Do not put any code in this frame.\n(It is a separator no-op. You can make a copy of this frame to create a new Macro frame)"
        n157 = Unbundle By Name(w433) -> ("Instrument UI.Lockin"=w427:refnum<class "Instrument UI.Lockin.lvclass">, "Instrument.Lockin"=w428:refnum<class "Instrument.Lockin.lvclass">)
        n158 = call <userlib>:"Create UI.vi"("error in (no error)"=w429, "Instrument in"=w428, "Instrument UI"=w427) -> ("error out"=w430:errorcluster, "Instrument UI out"=w431:refnum<class "Instrument UI.Lockin.lvclass">)  [unwired: 7 in]
        n159 = Bundle By Name(cluster=w433, "Instrument UI.Lockin"=w431) -> (w432:T5)
        n160 = call <vilib>:"Add State(s) to Queue__jki_lib_state_machine.vi"("State(s) in (\"\")"=w436) -> ("States Out"=w435:string)  [unwired: 14 in]
      }
      frame "SMO: Start Instrument UI" {
        # "Do not put any code in this frame.\n(It is a separator no-op. You can make a copy of this frame to create a new Macro frame)"
        n161 = Unbundle By Name(w440) -> ("Instrument UI.Lockin"=w439:refnum<class "Instrument UI.Lockin.lvclass">)
        n162 = call <vilib>:"Start.vi"("error in (no error)"=w438, "SMO"=w439) -> ("error out"=w437:errorcluster)  [unwired: 8 in, 1 out]
        n163 = call <vilib>:"Add State(s) to Queue__jki_lib_state_machine.vi"("State(s) in (\"\")"=w443) -> ("States Out"=w442:string)  [unwired: 14 in]
      }
      frame "SMO: Show Instrument UI" {
        # "Do not put any code in this frame.\n(It is a separator no-op. You can make a copy of this frame to create a new Macro frame)"
        n164 = Unbundle By Name(w451) -> ("Instrument UI.Lockin"=w449:refnum<class "Instrument UI.Lockin.lvclass">)
        n165 = call <vilib>:"GetState.vi"("error in (no error)"=w447, "SMO"=w449) -> ("error out"=w445:errorcluster, "SMO State"=w444:T1, "SMO out"=w448:refnum<class "Instrument UI.Lockin.lvclass">)  [unwired: 7 in]
        n166 = call <vilib>:"Clear Errors.vi"("error in (no error)"=w445) -> ("error out"=w446:errorcluster)  [unwired: 5 in, 1 out]
        n167 = case shown="\"Started\"" w444 {
          tunnel: [w455 w458] -> w450
          tunnel: w448 -> [_ w457]
          tunnel: w446 -> [w455 w456]
          frame Default {
          }
          frame "Started" {
            n168 = call <vilib>:"Show.vi"("error in (no error)"=w456, "SMO.UI"=w457) -> ("error out"=w458:errorcluster)  [unwired: 8 in, 1 out]
          }
        }
        n169 = call <vilib>:"Add State(s) to Queue__jki_lib_state_machine.vi"("State(s) in (\"\")"=w454) -> ("States Out"=w453:string)  [unwired: 14 in]
      }
      frame "SMO: Hide Instrument UI" {
        # "Do not put any code in this frame.\n(It is a separator no-op. You can make a copy of this frame to create a new Macro frame)"
        n170 = Unbundle By Name(w466) -> ("Instrument UI.Lockin"=w464:refnum<class "Instrument UI.Lockin.lvclass">)
        n171 = call <vilib>:"GetState.vi"("error in (no error)"=w462, "SMO"=w464) -> ("error out"=w460:errorcluster, "SMO State"=w459:T1, "SMO out"=w463:refnum<class "Instrument UI.Lockin.lvclass">)  [unwired: 7 in]
        n172 = call <vilib>:"Clear Errors.vi"("error in (no error)"=w460) -> ("error out"=w461:errorcluster)  [unwired: 5 in, 1 out]
        n173 = case shown="Default" w459 {
          tunnel: [w470 w473] -> w465
          tunnel: w463 -> [_ w472]
          tunnel: w461 -> [w470 w471]
          frame Default {
          }
          frame "Started" {
            n174 = call <vilib>:"Hide.vi"("error in (no error)"=w471, "SMO.UI"=w472) -> ("error out"=w473:errorcluster)  [unwired: 8 in, 1 out]
          }
        }
        n175 = call <vilib>:"Add State(s) to Queue__jki_lib_state_machine.vi"("State(s) in (\"\")"=w469) -> ("States Out"=w468:string)  [unwired: 14 in]
      }
      frame "SMO: Stop Instrument UI" {
        # "Do not put any code in this frame.\n(It is a separator no-op. You can make a copy of this frame to create a new Macro frame)"
        n176 = Unbundle By Name(w480) -> ("Instrument UI.Lockin"=w475:refnum<class "Instrument UI.Lockin.lvclass">)
        n177 = call <vilib>:"GetState.vi"("error in (no error)"=w479, "SMO"=w475) -> ("error out"=w478:errorcluster, "SMO State"=w476:T1, "SMO out"=w474:refnum<class "Instrument UI.Lockin.lvclass">)  [unwired: 7 in]
        n178 = call <vilib>:"Clear Errors.vi"("error in (no error)"=w478) -> ("error out"=w477:errorcluster)  [unwired: 5 in, 1 out]
        n179 = case shown="\"Created\", \"Started\"" w476 {
          tunnel: [w485 w488] -> w481
          tunnel: w474 -> [_ w487]
          tunnel: w477 -> [w485 w486]
          frame Default {
          }
          frame "Created", "Started" {
            n180 = call <vilib>:"Stop.vi"("error in (no error)"=w486, "SMO"=w487) -> ("error out"=w488:errorcluster)  [unwired: 8 in, 1 out]
          }
        }
        n181 = call <vilib>:"Add State(s) to Queue__jki_lib_state_machine.vi"("State(s) in (\"\")"=w484) -> ("States Out"=w483:string)  [unwired: 14 in]
      }
      frame "SMO: Destroy Instrument UI" {
        # "Do not put any code in this frame.\n(It is a separator no-op. You can make a copy of this frame to create a new Macro frame)"
        n182 = Unbundle By Name(w495) -> ("Instrument UI.Lockin"=w494:refnum<class "Instrument UI.Lockin.lvclass">)
        n183 = call <vilib>:"GetState.vi"("error in (no error)"=w492, "SMO"=w494) -> ("error out"=w491:errorcluster, "SMO State"=w489:T1, "SMO out"=w493:refnum<class "Instrument UI.Lockin.lvclass">)  [unwired: 7 in]
        n184 = call <vilib>:"Clear Errors.vi"("error in (no error)"=w491) -> ("error out"=w490:errorcluster)  [unwired: 5 in, 1 out]
        n185 = case shown="\"Stopped\"" w489 {
          tunnel: w490 -> [w500 w503]
          tunnel: [w500 w502] -> w496
          tunnel: w493 -> [_ w501]
          frame Default {
          }
          frame "Stopped" {
            n186 = call <vilib>:"Destroy.vi"("error in (no error)"=w503, "SMO"=w501) -> ("error out"=w502:errorcluster)  [unwired: 9 in]
          }
        }
        n187 = call <vilib>:"Add State(s) to Queue__jki_lib_state_machine.vi"("State(s) in (\"\")"=w499) -> ("States Out"=w498:string)  [unwired: 14 in]
      }
      frame "---------- Splash ----------" {
        # "Template Separator\n(You can make a copy of, or modify, this frame)"
        n188 = call <vilib>:"Add State(s) to Queue__jki_lib_state_machine.vi"("State(s) in (\"\")"=w508) -> ("States Out"=w507:string)  [unwired: 14 in]
      }
      frame "Splash: Set Status" {
        # "Your code here.\n(You can make a copy of, or modify, this frame)"
        n189 = property on="Splash Status" class="Str"(error in=w511, "Value"=w512) -> (error out=w510:errorcluster)  [unwired: 1 in, 1 out]
        n190 = call <vilib>:"Add State(s) to Queue__jki_lib_state_machine.vi"("State(s) in (\"\")"=w515) -> ("States Out"=w514:string)  [unwired: 14 in]
      }
      frame "Splash: 2" {
        # "Your code here.\n(You can make a copy of, or modify, this frame)"
        n191 = call <vilib>:"Add State(s) to Queue__jki_lib_state_machine.vi"("State(s) in (\"\")"=w520) -> ("States Out"=w519:string)  [unwired: 14 in]
      }
    }
  }
  "error out" <- w1
